vi "Process Controls.vi"(8 "error in (no error)":errorcluster {"code" format="Error %.0f"}, 10 "Controls":refnum<class "GUI Documentation.lvclass">[](array[class]), 11 "VIDoc Printer In":refnum<class "VIDoc Printer.lvclass">) -> (0 "error out":errorcluster {"code" format="Error %.0f"}, 3 "VIDoc Printer Out":refnum<class "VIDoc Printer.lvclass">)   [LabVIEW 2023, in "VIDoc Printer.lvlib" / "VIDoc Printer.lvclass"]
uses:
  VIDoc Printer.lvclass
  Parsing/GUI Documentation/GUI Documentation.lvclass
  VIDoc Printer.lvclass/VIDoc Printer.ctl
  Accessors/Get Controls Enabled.vi
  Accessors/Process Actions/Get Process Control Actions.vi
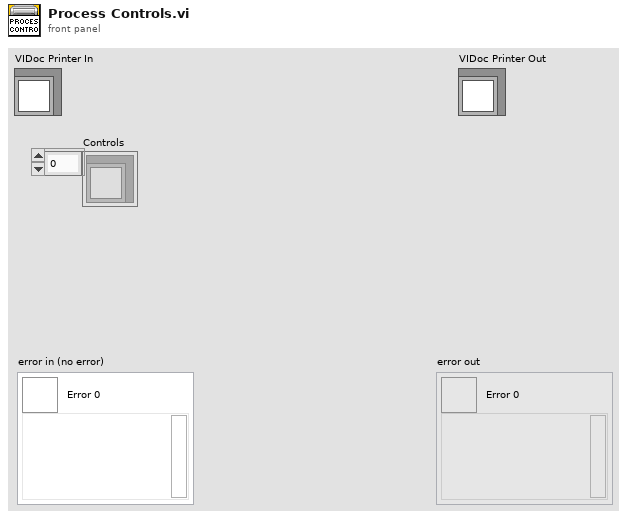
[diagram p1: front panel]
types:
  T1 = typedef "VIDoc Printer.lvlib/VIDoc Printer.lvclass/Process Control Enum.ctl" = enum16{"Header", "Memory", "By Folder", "By Tree", "By List", "Controls"}
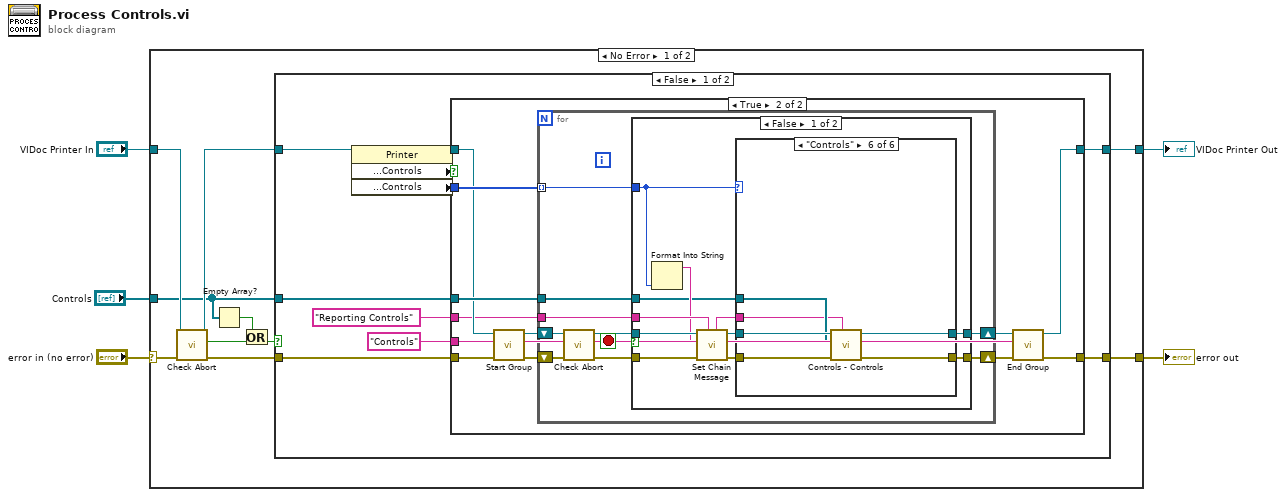
[diagram p0: block diagram]
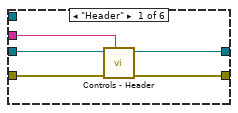
[diagram p3: hidden frame]
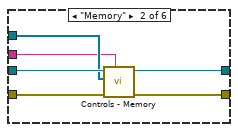
[diagram p4: hidden frame]
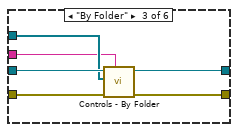
[diagram p5: hidden frame]
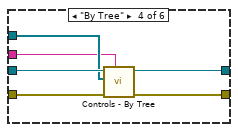
[diagram p6: hidden frame]
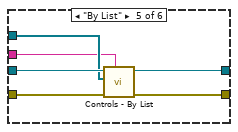
[diagram p7: hidden frame]
diagram:
  n1 = case shown="No Error" "error in (no error)" {
    selector: "error in (no error)" -> [w15 w101]
    tunnel: [w10 w101] -> w4
    tunnel: [w9 w100] -> w2
    tunnel: "VIDoc Printer In" -> [w12 w100]
    tunnel: "Controls" -> [w8 _]
    frame No Error {
      n2 = call "Check Abort.vi"("error in (no error)"=w15, "VIDoc Printer In"=w12) -> ("error out"=w14:errorcluster, "Abort?"=w11:bool, "VIDoc Printer Out"=w13:refnum<class "VIDoc Printer.lvclass">)  [unwired: 7 in]
      n3 = Empty Array?(array=w8) -> (empty?=w6:bool)
      n4 = Or(x=w6, y=w11) -> (x .or. y?=w7:bool)
      n5 = case shown="False" w7 {
        tunnel: w8 -> [w25 _]
        tunnel: w14 -> [w22 w99]
        tunnel: w13 -> [w23 w98]
        tunnel: [w20 w99] -> w10
        tunnel: [w21 w98] -> w9
        frame False {
          n6 = property class="Printer"(reference=w23) -> (reference out=w24:refnum<class "VIDoc Printer.lvclass">, "Properties:Settings:Enabled Sections:Controls"=w17:bool, "Properties:Process Lists:Controls"=w16:T1[])  [unwired: 1 in, 1 out]
          n7 = case shown="True" w17 {
            tunnel: w22 -> [w27 w37]
            tunnel: "Reporting Controls" ("string") -> [_ w29]
            tunnel: [w27 w30] -> w20
            tunnel: w25 -> [_ w39]
            tunnel: w24 -> [w26 w34]
            tunnel: [w26 w31] -> w21
            tunnel: w16 -> [_ w38]
            tunnel: "Controls" ("string") -> [_ w28]
            frame False {
            }
            frame True {
              n8 = call-dynamic "Start Group.vi"("error in (no error)"=w37, "Group"=w28, "VIDoc Printer In"=w34) -> ("error out"=w36:errorcluster, "VIDoc Printer Out"=w35:refnum<class "VIDoc Printer.lvclass">)  [unwired: 7 in]
              n9 = for {
                shift-right: [w47] -> w32
                shift-left: w36 -> [w49]
                tunnel: w29 -> [w43]
                tunnel: w39 -> [w42]
                shift-right: [w45] -> w33
                shift-left: w35 -> [w48]
                tunnel: w38 -> [w41] mode=indexing
                stop <- w40 stop-if-true
                n10 = call "Check Abort.vi"("error in (no error)"=w49, "VIDoc Printer In"=w48) -> ("error out"=w46:errorcluster, "Abort?"=w40:bool, "VIDoc Printer Out"=w44:refnum<class "VIDoc Printer.lvclass">)  [unwired: 7 in]
                n11 = case shown="False" w40 {
                  tunnel: [w60 w97] -> w47
                  tunnel: w46 -> [w57 w97]
                  tunnel: [w59 w96] -> w45
                  tunnel: w44 -> [w55 w96]
                  tunnel: w43 -> [w54 _]
                  tunnel: w42 -> [w51 _]
                  tunnel: w41 -> [w53 _]
                  frame False {
                    n12 = Format Into String(w53) -> (resulting string=w52:string)  [unwired: 3 in, 1 out]
                    n13 = call "Set Chain Message.vi"("Msg Chain"=w54, "error in (no error)"=w57, "New"=w52, "VIDoc Printer In"=w55) -> ("error out"=w58:errorcluster, "VIDoc Printer Out"=w56:refnum<class "VIDoc Printer.lvclass">, "Msg Chain out"=w50:string)  [unwired: 5 in]
                    n14 = case shown="\"Controls\"" w53 {
                      tunnel: w58 -> [w64 w70 w76 w82 w88 w94]
                      tunnel: [w62 w68 w74 w80 w86 w92] -> w60
                      tunnel: w56 -> [w65 w71 w77 w83 w89 w95]
                      tunnel: [w63 w69 w75 w81 w87 w93] -> w59
                      tunnel: w51 -> [_ w67 w73 w79 w85 w91]
                      tunnel: w50 -> [w61 w66 w72 w78 w84 w90]
                      frame "Header" {
                        n15 = call-dynamic "Controls - Header.vi"("Msg Chain"=w61, "error in (no error)"=w64, "VIDoc Printer In"=w65) -> ("error out"=w62:errorcluster, "VIDoc Printer Out"=w63:refnum<class "VIDoc Printer.lvclass">)  [unwired: 7 in]
                      }
                      frame "Memory" {
                        n16 = call-dynamic "Controls - Memory.vi"("Msg Chain"=w66, "error in (no error)"=w70, "Controls Docs"=w67, "VIDoc Printer In"=w71) -> ("error out"=w68:errorcluster, "VIDoc Printer Out"=w69:refnum<class "VIDoc Printer.lvclass">)  [unwired: 6 in]
                      }
                      frame "By Folder" {
                        n17 = call-dynamic "Controls - By Folder.vi"("Msg Chain"=w72, "error in (no error)"=w76, "Controls Docs"=w73, "VIDoc Printer In"=w77) -> ("error out"=w74:errorcluster, "VIDoc Printer Out"=w75:refnum<class "VIDoc Printer.lvclass">)  [unwired: 6 in]
                      }
                      frame "By Tree" {
                        n18 = call-dynamic "Controls - By Tree.vi"("Msg Chain"=w78, "error in (no error)"=w82, "Controls Docs"=w79, "VIDoc Printer In"=w83) -> ("error out"=w80:errorcluster, "VIDoc Printer Out"=w81:refnum<class "VIDoc Printer.lvclass">)  [unwired: 6 in]
                      }
                      frame "By List" {
                        n19 = call-dynamic "Controls - By List.vi"("Msg Chain"=w84, "error in (no error)"=w88, "Controls Docs"=w85, "VIDoc Printer In"=w89) -> ("error out"=w86:errorcluster, "VIDoc Printer Out"=w87:refnum<class "VIDoc Printer.lvclass">)  [unwired: 6 in]
                      }
                      frame "Controls" {
                        n20 = call-dynamic "Controls - Controls.vi"("Msg Chain"=w90, "error in (no error)"=w94, "Controls Docs"=w91, "VIDoc Printer In"=w95) -> ("error out"=w92:errorcluster, "VIDoc Printer Out"=w93:refnum<class "VIDoc Printer.lvclass">)  [unwired: 6 in]
                      }
                    }
                  }
                  frame True {
                  }
                }
              }
              n21 = call-dynamic "End Group.vi"("error in (no error)"=w32, "Group"=w28, "VIDoc Printer In"=w33) -> ("error out"=w30:errorcluster, "VIDoc Printer Out"=w31:refnum<class "VIDoc Printer.lvclass">)  [unwired: 7 in]
            }
          }
        }
        frame True {
        }
      }
    }
    frame Error {
    }
  }
  "error out" <- w4
  "VIDoc Printer Out" <- w2
